vi "Check Dirty.vi"(8 "error in (no error)":errorcluster, 11 "GitPackage in":refnum<class "GitPackage.lvclass">) -> (0 "error out":errorcluster, 2 "Dirty":bool, 3 "GitPackage out":refnum<class "GitPackage.lvclass">)   [LabVIEW 2020, in "GPack.lvlib" / "GitPackage.lvclass"]
uses:
  GitPackage.lvclass
  <vilib>/Utility/error.llb/whitespace.ctl
  GitPackage.lvclass/GitPackage.ctl
  <vilib>/Hampel Software Engineering/Git API/Git API/GIT-api.lvclass/GIT-api.ctl
  <vilib>/Hampel Software Engineering/Git API/Git API/GIT-api.lvclass
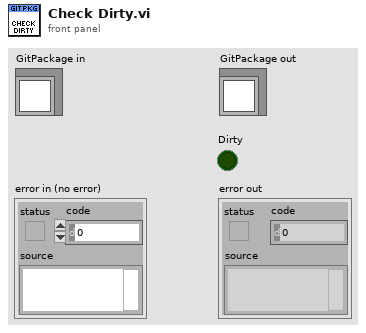
[diagram p1: front panel]
types:
  T1 = typedef "whitespace.ctl" = u16
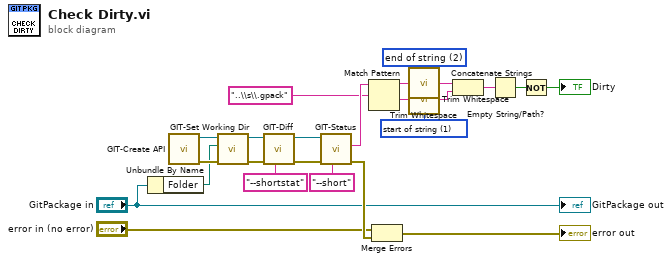
[diagram p0: block diagram]
diagram:
  w6 = T1 1 items=["both", "start of string", "end of string"] ("location (both)")
  w8 = T1 2 items=["both", "start of string", "end of string"] ("location (both)")
  n1 = Unbundle By Name("GitPackage in") -> ("Folder"=w12:path)
  n2 = call <vilib>:"GIT-Create API.vi"() -> ("error out"=w23:errorcluster, "git-api out"=w21:refnum<class "GIT-api.lvclass">)  [unwired: 10 in]
  n3 = call <vilib>:"GIT-Set Working Dir.vi"("error in"=w23, "Working Directory"=w12, "git-api in"=w21) -> ("error out"=w15:errorcluster, "git-api out"=w19:refnum<class "GIT-api.lvclass">)  [unwired: 7 in]
  n4 = call <vilib>:"GIT-Diff.vi"("param"="--shortstat", "error in"=w15, "git-api in"=w19) -> ("error out"=w14:errorcluster, "git-api out"=w17:refnum<class "GIT-api.lvclass">)  [unwired: 6 in, 1 out]
  n5 = call <vilib>:"GIT-Status.vi"("param"="--short", "error in"=w14, "git-api in"=w17) -> ("error out"=w24:errorcluster, "std out"=w11:string)  [unwired: 6 in, 1 out]
  n6 = Match Pattern(string=w11, regular expression="..\\s\\.gpack") -> (before substring=w9:string, after substring=w7:string)  [unwired: 1 in, 2 out]
  n7 = Merge Errors("error in (no error)", w24) -> (→"error out":errorcluster)
  n8 = call <vilib>:"Trim Whitespace.vi"("string"=w9, "location (both)"=w8) -> ("trimmed string"=w5:string)
  n9 = call <vilib>:"Trim Whitespace.vi"("string"=w7, "location (both)"=w6) -> ("trimmed string"=w4:string)
  n10 = Concatenate Strings(w5, w4) -> (w3:string)
  n11 = Empty String/Path?(string/path=w3) -> (empty?=w2:bool)
  n12 = Not(x=w2) -> (.not. x?=→"Dirty":bool)
  "GitPackage out" <- "GitPackage in"
